vi "Write Interface protocol.vi"(10 "Interface protocol":T1(ring), 11 "Device in":refnum<class "PIC-Device.lvclass">) -> (3 "Device out":refnum<class "PIC-Device.lvclass">)   [LabVIEW 2020, in "PIC-Device.lvclass"]
uses:
  PIC-Device.lvclass
  PIC-Device.lvclass/PIC-Device.ctl
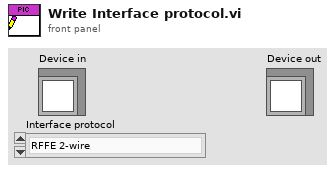
[diagram p1: front panel]
types:
  T1 = enum16{"RFFE 2-wire", "WiSPI 3-wire spi_sel", "WiSPI 4-wire spi_sel", "ifxSPI 3-wire spi_sel", "WiSPI 3-wire dev add spi_sel"}
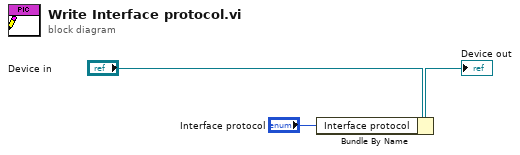
[diagram p0: block diagram]
diagram:
  n1 = Bundle By Name(cluster="Device in", "Interface protocol"="Interface protocol") -> (→"Device out":refnum<class "PIC-Device.lvclass">)
